vi "Get Setpoints.vi"(11 "Task Actor in":refnum<class "Task Actor.lvclass">) -> (2 "Setpoints":T1(c390), 3 "Task Actor out":refnum<class "Task Actor.lvclass">)   [LabVIEW 2024, in "Task Actor.lvlib" / "Task Actor.lvclass"]
uses:
  Task Actor.lvclass
  Task Actor.lvclass/Task Actor.ctl
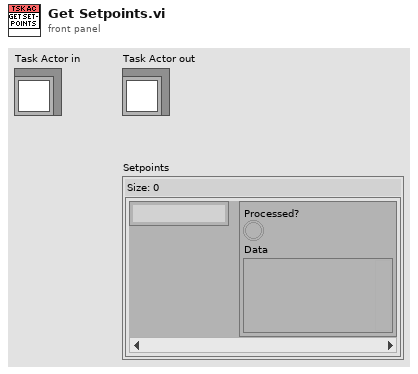
[diagram p1: front panel]
types:
  T1 = map{string, cluster{"Processed?":bool, "Data":variant}}
  T2 = map{string, cluster{"New?":bool, "Data":variant}}
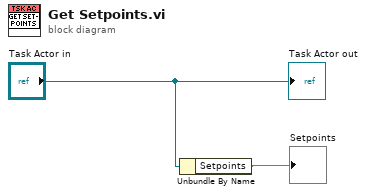
[diagram p0: block diagram]
diagram:
  n1 = Unbundle By Name("Task Actor in") -> ("Setpoints"=→"Setpoints":T2)
  "Task Actor out" <- "Task Actor in"
